vi "filtroButterworthLowpass.vi"(1 "element":u32) -> (0 "Filtered X":dbl[](array[numeric]))   [LabVIEW 2013]
uses:
  <vilib>/Analysis/3filter.llb/Filter Passband Type.ctl
  <vilib>/Analysis/3filter.llb/Butterworth Filter (DBL).vi
  <vilib>/Analysis/NI_AALBase.lvlib
panel:
  in  "filterData":u32[](array[numeric])
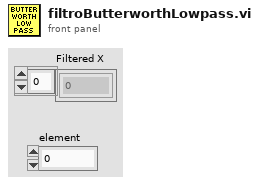
[diagram p1: front panel]
types:
  T1 = typedef "NI_AALBase.lvlib/Filter Passband Type.ctl" = enum32{"Lowpass", "Highpass", "Bandpass", "Bandstop"}
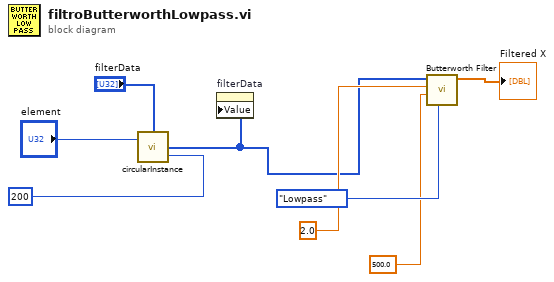
[diagram p0: block diagram]
diagram:
  n1 = call "circularInstance.vi"("data"="filterData", "max-size"=i16 200, "element"="element") -> ("dataout"=w4:u32[])
  n2 = property on="filterData" class="Arr (strict)"("Value"=w4) -> ()  [unwired: 2 in, 2 out]
  n3 = call-poly <vilib>:"Butterworth Filter.vi"("filter type"=Filter_Passband_Type."Lowpass", "high cutoff freq: fh"=500.0, "sampling freq: fs"=2.0, "X"=w4) -> ("Filtered X"=→"Filtered X":dbl[])  [unwired: 4 in, 1 out]
